vi "Table_ScrollaBarMarvin.vi"(3 "error in":errorcluster, 4 "Line to focus":string, 6 "TableIn":refnum<vi>) -> (0 "error out":errorcluster, 1 "reference out":refnum<vi>, 5 "OK?":bool)   [LabVIEW 2017]
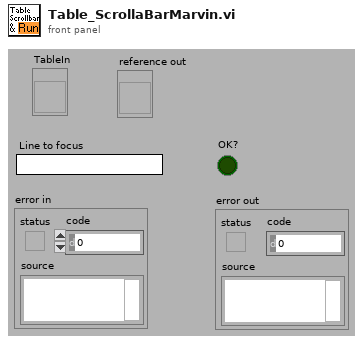
[diagram p1: front panel]
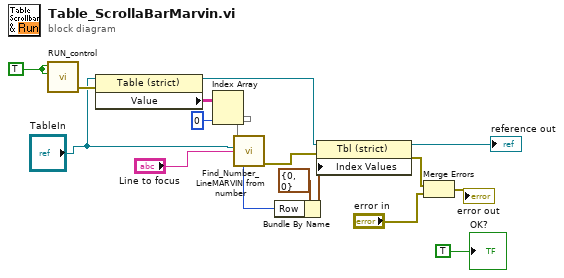
[diagram p0: block diagram]
diagram:
  w5 = TRUE ("Blinking")
  n1 = call "RUN_control.vi"("Blinking(:T)"=w5, "Value (:T)"=w5) -> ("error out"=w6:errorcluster)  [unwired: 3 in, 2 out]
  n2 = property on="Property Node" class="Table (strict)"(reference="TableIn", error in=w6) -> (reference out=w7:refnum<vi>, "Value"=w3:string[][])  [unwired: 1 out]
  n3 = Index Array(array=w3, index (col)=0 ("disabled index (col)")) -> (element=w2:string[])  [unwired: 1 in]
  n4 = call "Find_Number_LineMARVIN from number.vi"("Test Paragraph"="Line to focus", "TableIn"="TableIn", "Row Headers[]"=w2) -> ("error out"=w13:errorcluster, "Line number"=w15:i32)  [unwired: 2 in, 2 out]
  n5 = Bundle By Name(cluster=cluster{"Row":i32, "Column":i32} {"Row"=0, "Column"=0} ("Edit Position"), "Row"=w15) -> (w16:cluster{"Row":i32, "Column":i32})
  n6 = property on="Property Node" class="Tbl (strict)"(reference=w7, error in=w13, "Index Values"=w16) -> (reference out=→"reference out":refnum<vi>, error out=w9:errorcluster)
  n7 = Merge Errors(w9, "error in") -> (→"error out":errorcluster)
  "OK?" <- TRUE ("OK?")
